vi "heaters.vi"() -> ()   [LabVIEW 2018]
uses:
  <vilib>/NI Modbus.llb/MB Serial Master Query Write Single Register (poly).vi
  <vilib>/NI Modbus.llb/MB Serial Master Query Write Multiple Registers (poly).vi
  <vilib>/NI Modbus.llb/MB Serial Master Query Read Holding Registers (poly).vi
  <vilib>/NI Modbus.llb/MB Serial Master Query Read Input Registers (poly).vi
panel:
  in  "milliseconds to wait":u32=1000
  out "PWM":u16[](array[numeric]) caption="PWM frequency"
  in  "PWM":u16 caption="PWM frequency"
  out "Input Registers":u16[](array[numeric]) caption="Total output load (%)"
  out "Holding Registers 2":u16[](array[numeric])
  in  "Serial Parameters":T1={"Mode"=enum."RTU", "Slave Address"=127}
  out "Bar 10":u16(slide) scale=0.0..100.0
  out "Bar 9":u16(slide) scale=0.0..100.0
  out "Bar 8":u16(slide) scale=0.0..100.0
  out "Bar 7":u16(slide) scale=0.0..100.0
  out "Bar 6":u16(slide) scale=0.0..100.0
  out "Bar 5":u16(slide) scale=0.0..100.0
  out "Bar 4":u16(slide) scale=0.0..100.0
  out "Bar 3":u16(slide) scale=0.0..100.0
  out "Bar 2":u16(slide) scale=0.0..100.0
  out "Bar":u16(slide) scale=0.0..100.0
  in  "stop":bool
  in  "Slide 20":u16(slide) scale=0.0..4095.0
  in  "Slide 19":u16(slide) scale=0.0..4095.0
  in  "Slide 18":u16(slide) scale=0.0..4095.0
  in  "Slide 17":u16(slide) scale=0.0..4095.0
  in  "Slide 16":u16(slide) scale=0.0..4095.0
  in  "Slide 15":u16(slide) scale=0.0..4095.0
  in  "Slide 14":u16(slide) scale=0.0..4095.0
  in  "Slide 13":u16(slide) scale=0.0..4095.0
  in  "Slide 12":u16(slide) scale=0.0..4095.0
  in  "Slide 11":u16(slide) scale=0.0..4095.0
  in  "Slide 10":u16(slide) scale=0.0..4095.0
  in  "Slide 9":u16(slide) scale=0.0..4095.0
  in  "Slide 8":u16(slide) scale=0.0..4095.0
  in  "Slide 7":u16(slide) scale=0.0..4095.0
  in  "Slide 6":u16(slide) scale=0.0..4095.0
  in  "Slide 5":u16(slide) scale=0.0..4095.0
  in  "Slide 4":u16(slide) scale=0.0..4095.0
  in  "Slide 3":u16(slide) scale=0.0..4095.0
  in  "Slide 2":u16(slide) scale=0.0..4095.0
  in  "Slide 1":u16(slide) scale=0.0..4095.0
  out "Holding Registers":u16[](array[numeric]) caption="Total load"
  in  "COM 3":refnum<visa-resource-name>
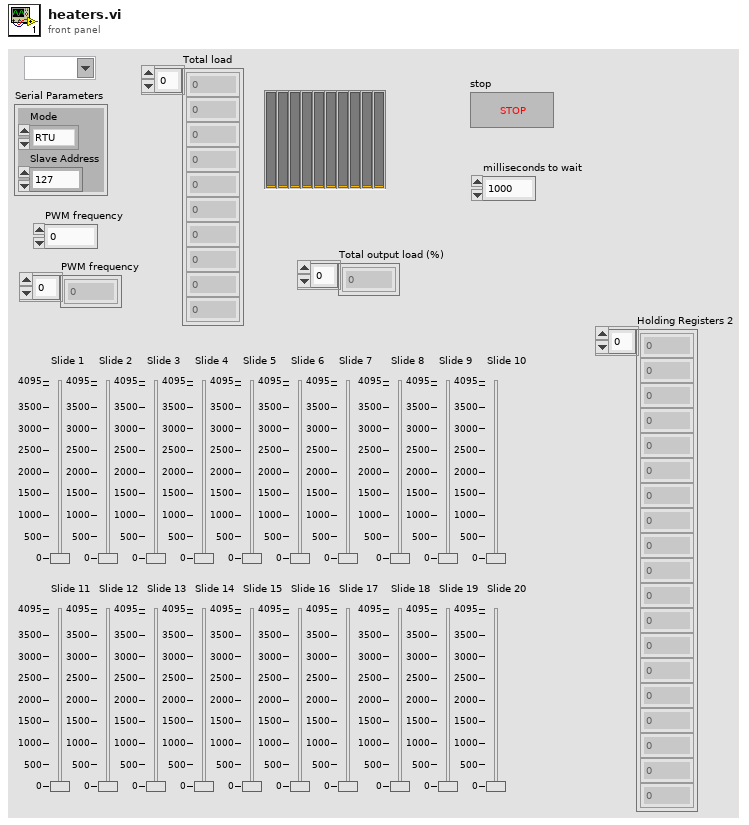
[diagram p1: front panel]
types:
  T1 = cluster{"Mode":enum16{"RTU", "ASCII"}, "Slave Address":u8}
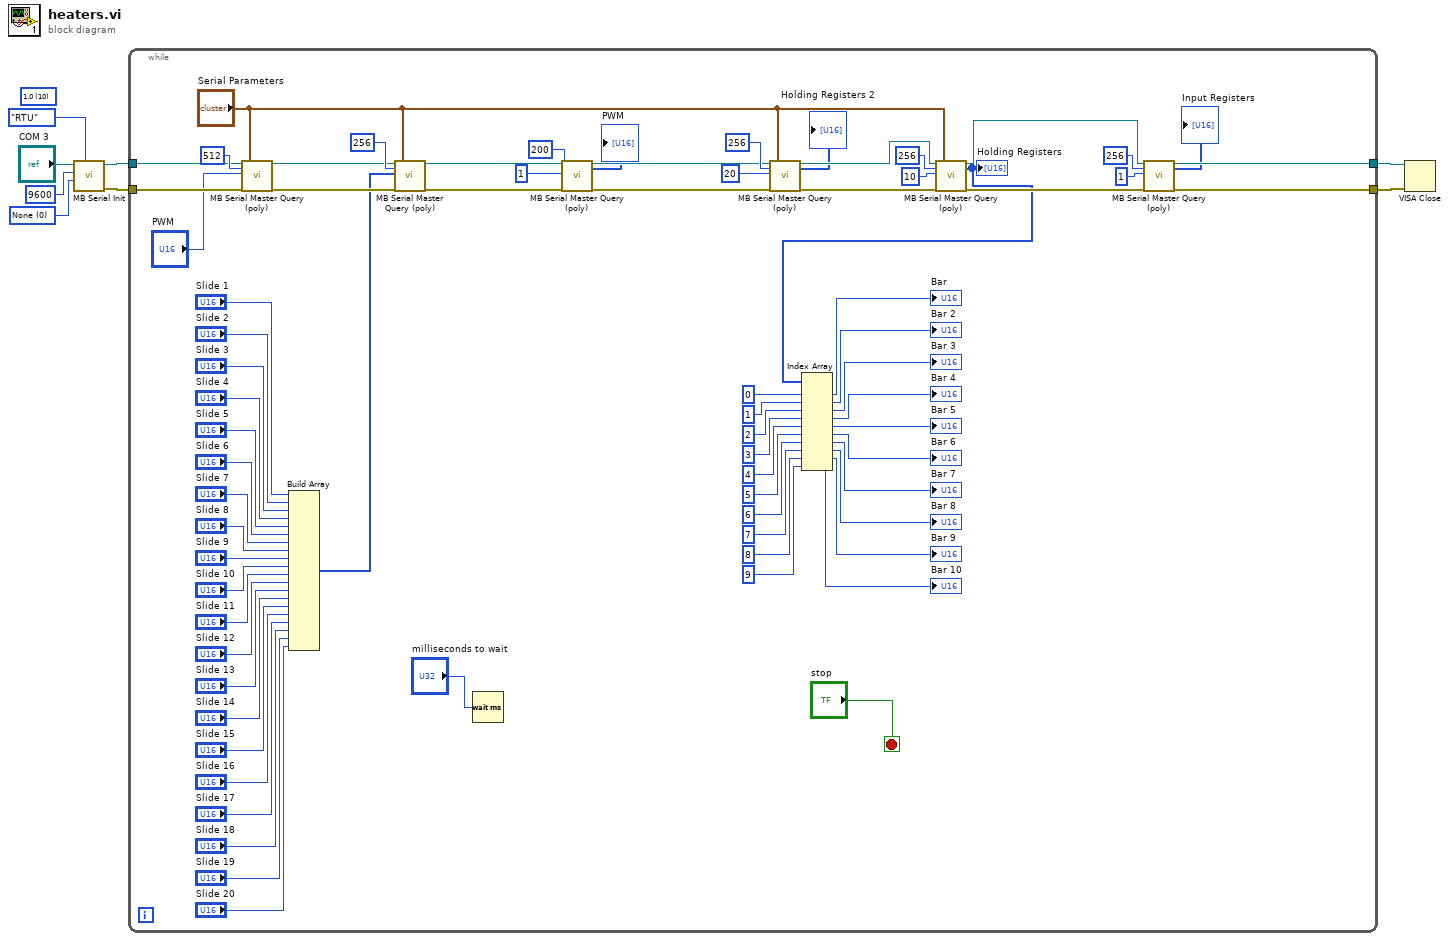
[diagram p0: block diagram]
diagram:
  (unwired) u16 10 items=["1.0"=10, "1.5"=15, "2.0"=20] ("Serial Settings:Serial Stop Bits")
  w7 = u16 0 items=["None", "Odd", "Even", "Mark", "Space"] ("Parity")
  n1 = call <vilib>:"MB Serial Init.vi"("Mode"=enum16{"RTU", "ASCII"}."RTU", "Parity"=w7, "Baud Rate"=u32 9600, "VISA resource name"="COM 3") -> ("error out"=w3:errorcluster, "VISA resource name out"=w4:refnum<visa-resource-name>)  [unwired: 6 in]
  n2 = while {
    tunnel: w4 -> [w79]
    tunnel: w3 -> [w78]
    tunnel: [w18] -> w2
    tunnel: [w77] -> w1
    stop <- "stop" stop-if-true
    n3 = call-poly <vilib>:"MB Serial Master Query (poly).vi"("VISA resource name"=w79, "Address"=u16 512, "Holding Register"="PWM", "error in"=w78, "Serial Parameters"="Serial Parameters") -> ("VISA resource name out"=w73:refnum<visa-resource-name>, "error out"=w72:errorcluster)  [unwired: 12 in, 1 out]
    n4 = Build Array("Slide 1", "Slide 2", "Slide 3", "Slide 4", "Slide 5", "Slide 6", "Slide 7", "Slide 8", "Slide 9", "Slide 10", "Slide 11", "Slide 12", "Slide 13", "Slide 14", "Slide 15", "Slide 16", "Slide 17", "Slide 18", "Slide 19", "Slide 20") -> (w51:u16[])
    n5 = call-poly <vilib>:"MB Serial Master Query (poly).vi"("VISA resource name"=w73, "Starting Address"=u16 256 ("Address"), "Registers"=w51, "error in"=w72, "Serial Parameters"="Serial Parameters") -> ("VISA resource name out"=w15:refnum<visa-resource-name>, "error out"=w13:errorcluster)  [unwired: 12 in, 1 out]
    n6 = Wait (ms)(milliseconds to wait="milliseconds to wait") -> ()  [unwired: 1 out]
    n7 = call-poly <vilib>:"MB Serial Master Query (poly).vi"("VISA resource name"=w15, "Starting Address"=u16 200, "Quantity"=u16 1, "error in"=w13) -> ("VISA resource name out"=w14:refnum<visa-resource-name>, "Holding Registers"=→"PWM":u16[], "error out"=w12:errorcluster)  [unwired: 12 in, 1 out]
    n8 = call-poly <vilib>:"MB Serial Master Query (poly).vi"("VISA resource name"=w14, "Starting Address"=u16 256 ("Address"), "Quantity"=u16 20, "error in"=w12, "Serial Parameters"="Serial Parameters") -> ("VISA resource name out"=w25:refnum<visa-resource-name>, "Holding Registers"=→"Holding Registers 2":u16[], "error out"=w26:errorcluster)  [unwired: 11 in, 1 out]
    n9 = call-poly <vilib>:"MB Serial Master Query (poly).vi"("VISA resource name"=w25, "Starting Address"=u16 256, "Quantity"=u16 10, "error in"=w26, "Serial Parameters"="Serial Parameters") -> ("VISA resource name out"=w19:refnum<visa-resource-name>, "Input Registers"=w36:u16[], "error out"=w77:errorcluster)  [unwired: 11 in, 1 out]
    "Holding Registers" <- w36
    n10 = Index Array(array=w36, index #1=0 ("index"), index #2=1 ("index"), index #3=2 ("index"), index #4=3 ("index"), index #5=4 ("index"), index #6=5 ("index"), index #7=6 ("index"), index #8=7 ("index"), index #9=8 ("index"), index #10=9 ("index")) -> (element #1=→"Bar":u16, element #2=→"Bar 2":u16, element #3=→"Bar 3":u16, element #4=→"Bar 4":u16, element #5=→"Bar 5":u16, element #6=→"Bar 6":u16, element #7=→"Bar 7":u16, element #8=→"Bar 8":u16, element #9=→"Bar 9":u16, element #10=→"Bar 10":u16)
    n11 = call-poly <vilib>:"MB Serial Master Query (poly).vi"("VISA resource name"=w19, "Starting Address"=u16 256, "Quantity"=u16 1) -> ("VISA resource name out"=w18:refnum<visa-resource-name>, "Input Registers"=→"Input Registers":u16[])  [unwired: 13 in, 2 out]
  }
  n12 = VISA Close(VISA resource name=w2, error in (no error)=w1) -> ()  [unwired: 1 out]
